vi "voltech4_test.vi"() -> ()   [LabVIEW 2015]
uses:
  <instrlib>/Voltech PM1000+/Voltech PM1000+.lvlib
  <vilib>/Utility/file.llb/Write To Spreadsheet File (string).vi
  <instrlib>/Voltech PM1000+/Public/Configure/Configure Measurements (Normal).vi
panel:
  out "error3":string
  out "output 3":string
  out "String 3":string
  out "output before loop":string
  out "error before":string
  in  "Minutes per test":dbl
  in  "FOLDER NAME":string
  in  "HOW MANY TEST":i32
  in  "Name of File":string
  in  "VISA resource name 2":refnum<visa-resource-name>
  out "Current Data Point":i32
  in  "stop":bool
  out "VRMS":dbl[](graph)
  in  "Normal Measurements":i32[](listbox)=[0, 1, 2, 3, 4, 5, 6]
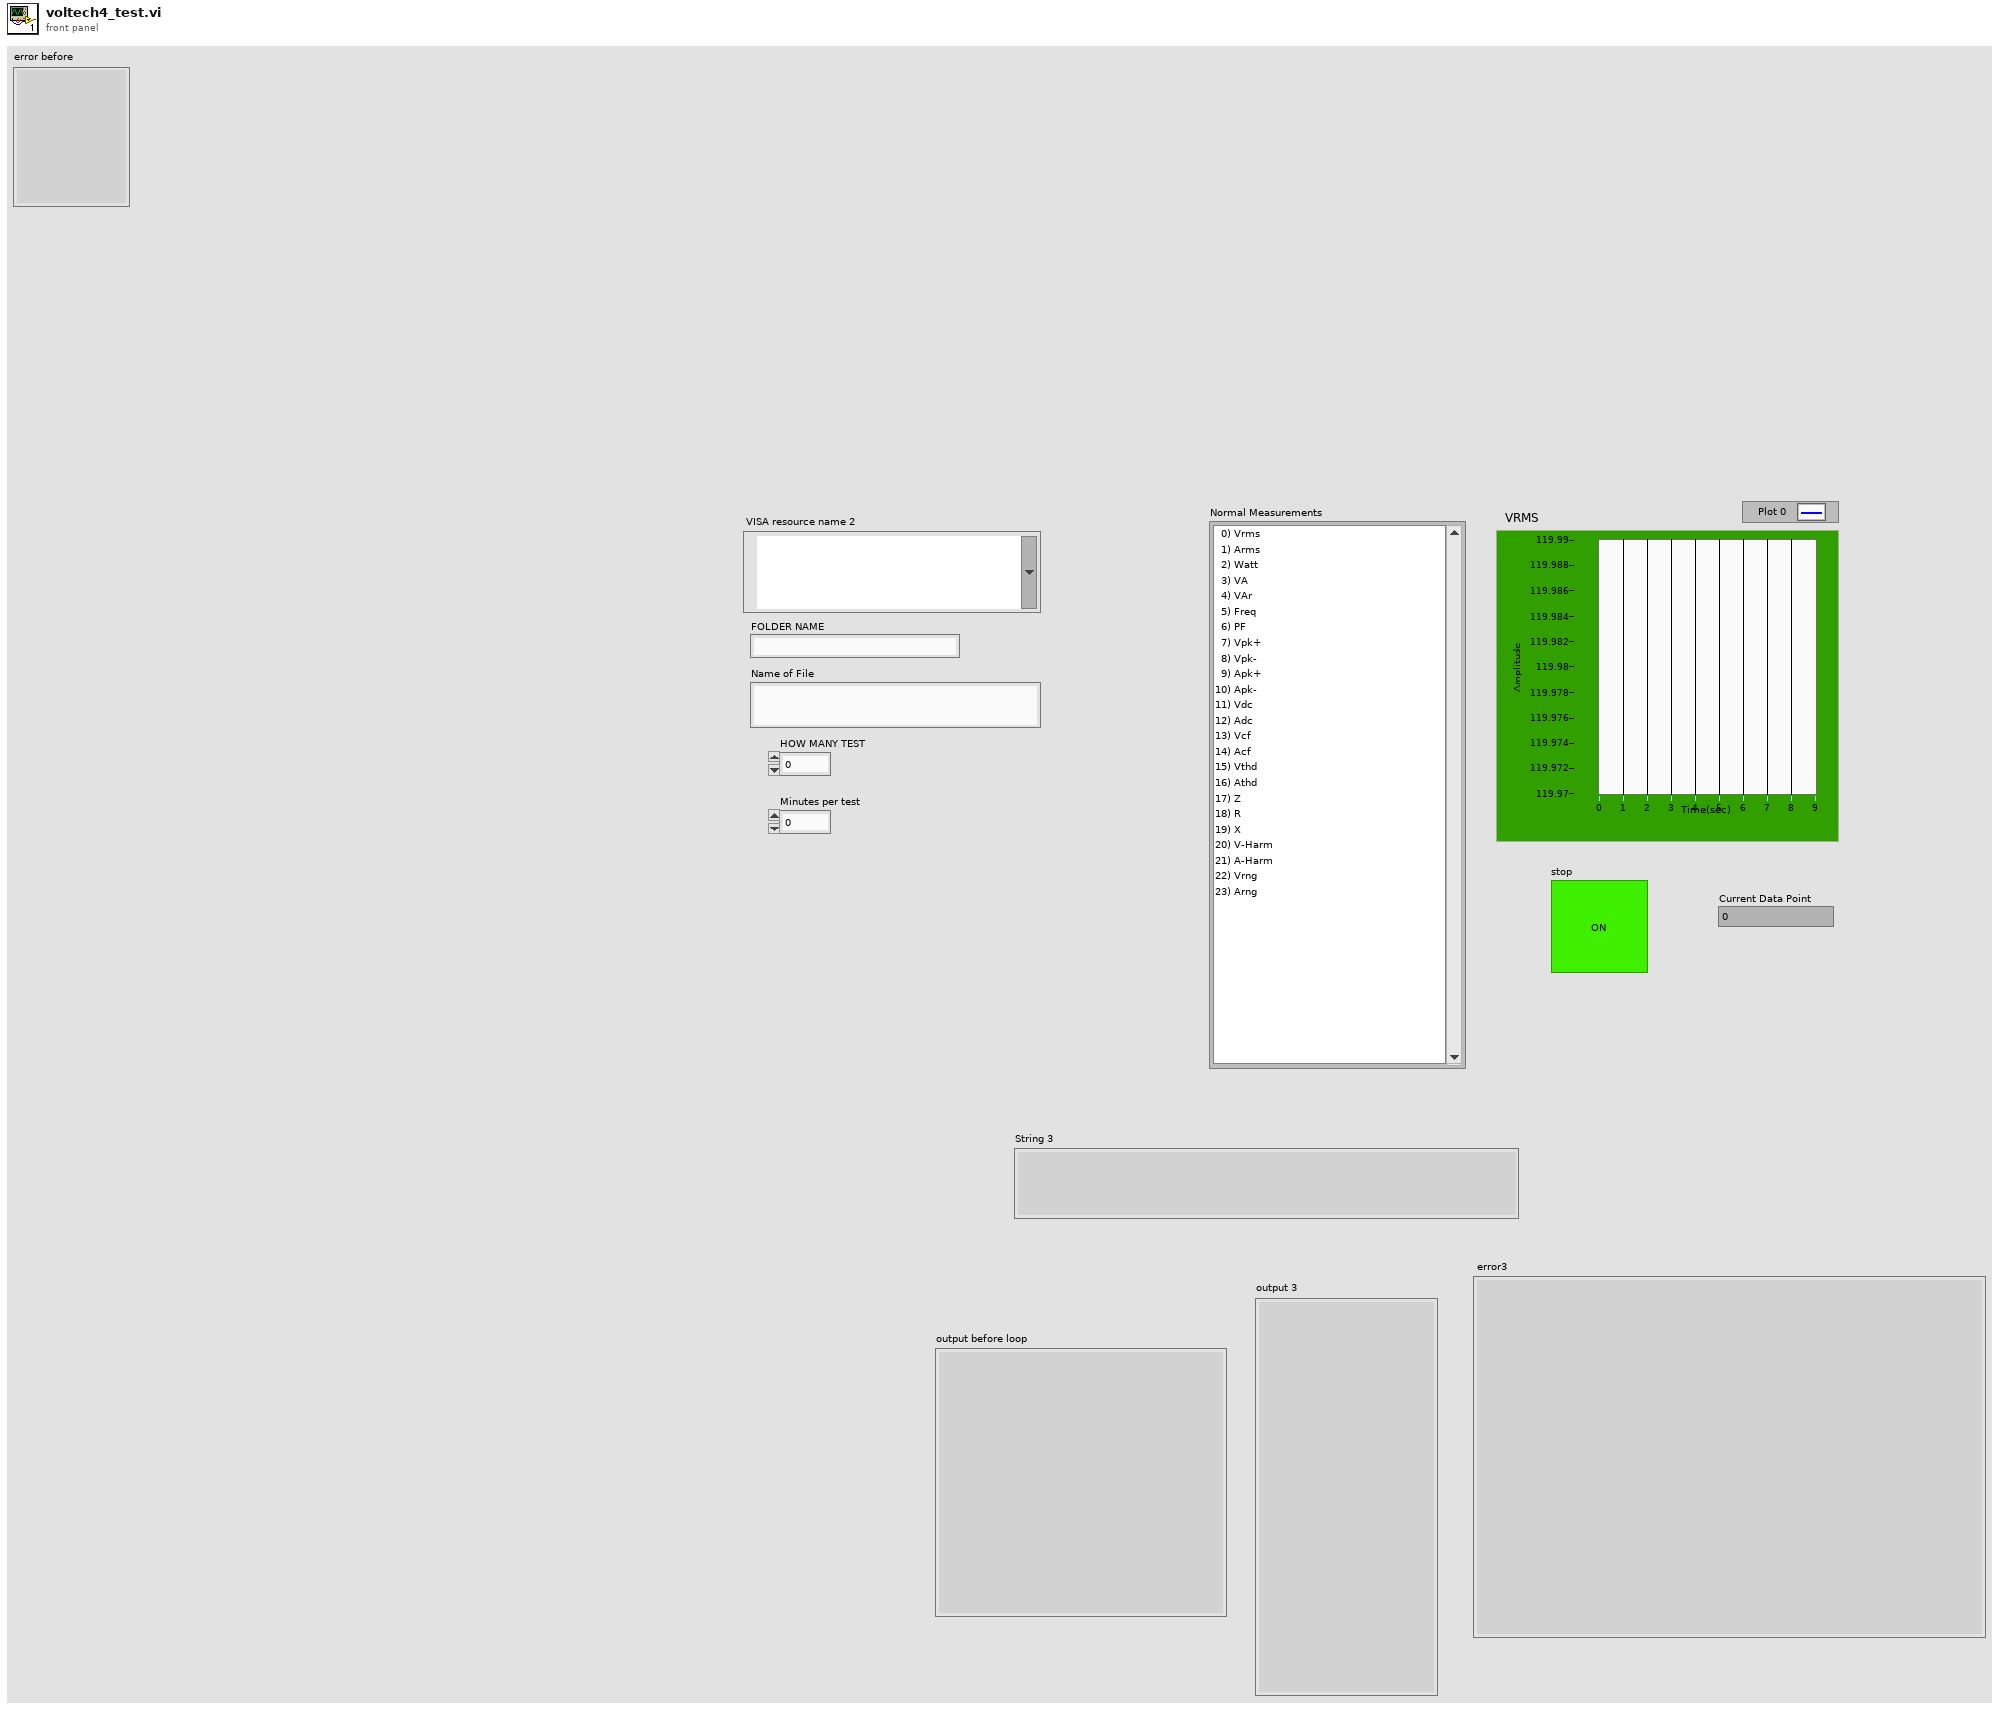
[diagram p1: front panel]
types:
  T1 = enum16{"open", "replace", "create", "open or create", "replace or create", "replace or create with confirmation"}
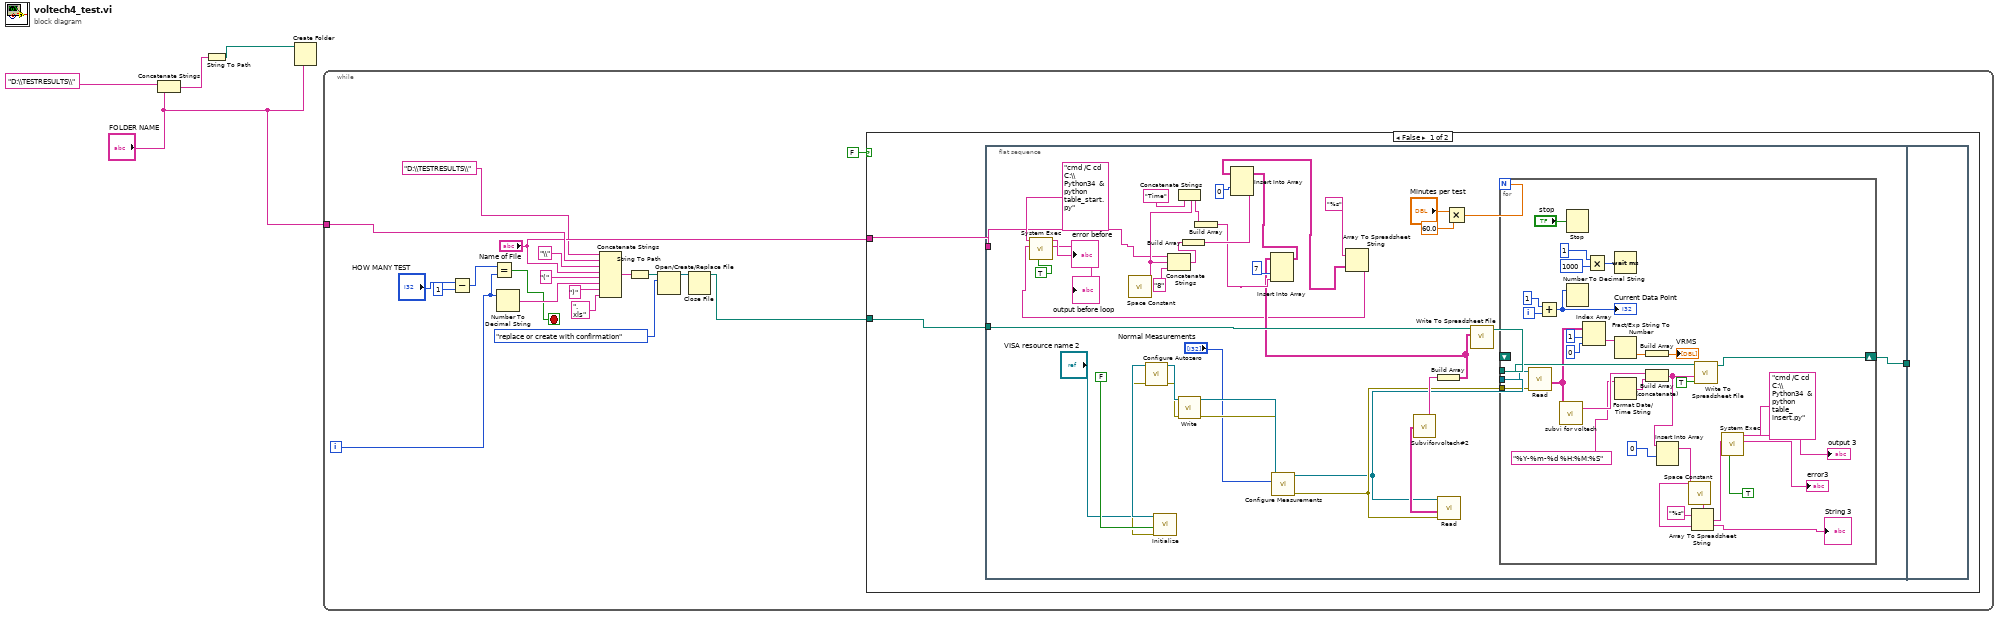
[diagram p0: block diagram]
diagram:
  n1 = Concatenate Strings("D:\\TESTRESULTS\\" ("string"), "FOLDER NAME") -> (w2:string)
  n2 = String To Path(string=w2) -> (path=w1:path)
  n3 = Create Folder(prompt (Create Folder)="FOLDER NAME", path (use dialog)=w1) -> ()  [unwired: 1 in, 3 out]
  n4 = while {
    tunnel: "FOLDER NAME" -> [w10]
    i -> [w11]
    stop <- w12 stop-if-true
    n5 = Subtract(x="HOW MANY TEST", y=1) -> (x-y=w7:i32)
    n6 = Equal?(x=w7, y=w11) -> (x = y?=w12:bool)
    n7 = Number To Decimal String(number=w11) -> (decimal integer string=w16:string)  [unwired: 1 in]
    n8 = Concatenate Strings("D:\\TESTRESULTS\\" ("string"), w10, "\\" ("string"), "Name of File", "(" ("string"), w16, ")" ("string"), ".xls" ("string")) -> (w20:string)
    n9 = String To Path(string=w20) -> (path=w21:path)
    n10 = Open/Create/Replace File(file path (use dialog)=w21, operation (0:open)=T1."replace or create with confirmation") -> (refnum out=w19:refnum<file>)  [unwired: 4 in, 2 out]
    n11 = Close File(refnum=w19) -> (path=w13:path)  [unwired: 1 in, 1 out]
    n12 = case shown="False" FALSE {
      tunnel: w13 -> [w26 _]
      tunnel: "Name of File" -> [w24 _]
      frame False {
        n13 = flat-sequence {
          tunnel: w26 -> [w54]
          tunnel: [w60] -> w25
          tunnel: w24 -> [w30]
          tunnel: w25 -> [_]
          frame #0 {
            n14 = call <vilib>:"Space Constant.vi"() -> ("String"=w35:string)
            n15 = call <instrlib>:"Initialize.vi"("Reset (True)"=FALSE, "VISA resource name"="VISA resource name 2") -> ("error out"=w62:errorcluster, "VISA resource name out"=w63:refnum<visa-resource-name>)  [unwired: 8 in]
            n16 = call <instrlib>:"Configure Autozero.vi"("error in (no error)"=w62, "VISA resource name"=w63) -> ("error out"=w58:errorcluster, "VISA resource name out"=w59:refnum<visa-resource-name>)  [unwired: 8 in]
            n17 = Concatenate Strings(w30, w35, "8") -> (w37:string)
            n18 = Concatenate Strings("Time", w35) -> (w32:string)
            n19 = call <instrlib>:"Write.vi"("error in (no error)"=w58, "VISA resource name"=w59) -> ("error out"=w56:errorcluster, "VISA resource name out"=w57:refnum<visa-resource-name>)  [unwired: 8 in]
            n20 = Build Array(w37) -> (w38:string[])
            n21 = Build Array(w32) -> (w33:string[])
            n22 = call-poly <instrlib>:"Configure Measurements.vi"("error in (no error)"=w56, "Normal Measurements"="Normal Measurements", "VISA resource name"=w57) -> ("error out"=w50:errorcluster, "VISA resource name out"=w49:refnum<visa-resource-name>)  [unwired: 7 in]
            n23 = call <instrlib>:"Read.vi"("error in (no error)"=w50, "VISA resource name"=w49) -> ("Measurement Results"=w51:string[][])  [unwired: 7 in, 2 out]
            n24 = call "Subviforvoltech#2.vi"("Measurement Results 2"=w51) -> ("Array"=w55:string[])
            n25 = Build Array(w55) -> (w29:string[][])
            n26 = Insert Into Array(array=w29, index (col)=7, new element=w33) -> (w40:string[][])  [unwired: 1 in]
            n27 = Insert Into Array(array=w40, index (col)=0, new element=w38) -> (w27:string[][])  [unwired: 1 in]
            n28 = Array To Spreadsheet String(array=w27, 3:"%s") -> (spreadsheet string=w28:string)  [unwired: 1 in]
            n29 = call <vilib>:"System Exec.vi"("run minimized? (F)"=TRUE, "standard input"=w28, "command line"="cmd /C cd C:\\Python34  & python table_start.py") -> ("standard error"=→"output before loop":string, "standard output"=→"error before":string)  [unwired: 5 in, 2 out]
            n30 = Multiply(x="Minutes per test", y=60.0) -> (x*y=w48:dbl)
            n31 = call-poly <vilib>:"Write To Spreadsheet File.vi"("2D data"=w29, "file path (dialog if empty)"=w54) -> ("new file path (Not A Path if cancelled)"=w53:path)  [unwired: 6 in]
            n32 = for {
              N: w48 -> [_]
              tunnel: w53 -> [w90]
              shift-right: [w88] -> w60
              shift-left: _ -> [_]
              tunnel: w49 -> [w86]
              tunnel: w50 -> [w85]
              i -> [w92]
              n33 = call <instrlib>:"Read.vi"("error in (no error)"=w85, "VISA resource name"=w86) -> ("Measurement Results"=w77:string[][])  [unwired: 7 in, 2 out]
              n34 = Add(x=1, y=w92) -> (x+y=w93:i32)
              "Current Data Point" <- w93
              n35 = call "subvi for voltech.vi"("Measurement Results 2"=w77) -> ("Array"=w87:string[])  [unwired: 6 in]
              n36 = Stop(stop? (T)="stop") -> ()
              n37 = Number To Decimal String(number=w93) -> ()  [unwired: 1 in, 1 out]
              n38 = Index Array(array=w77, index (row)=1, index (col)=0 ("disabled index (col)")) -> (element=w80:string)
              n39 = Multiply(x=u32 1 ("Interval of Data Collection (sec)"), y=u32 1000) -> (x*y=w94:u32)
              n40 = Wait (ms)(milliseconds to wait=w94) -> ()  [unwired: 1 out]
              n41 = Fract/Exp String To Number(string=w80) -> (number=w76:dbl)  [unwired: 3 in, 1 out]
              n42 = Format Date/Time String(time format string (%c)="%Y-%m-%d %H:%M:%S") -> (date/time string=w83:string)  [unwired: 2 in]
              n43 = Build Array(w76) -> (→"VRMS":dbl[])
              n44 = Build Array (concatenate)(w87, w83) -> (w68:string[])
              n45 = Insert Into Array(array=w68, index=0) -> (w73:string[])  [unwired: 1 in]
              n46 = call <vilib>:"Space Constant.vi"() -> ("String"=w75:string)
              n47 = Array To Spreadsheet String(delimiter (Tab)=w75, array=w73, 3:"%s") -> (spreadsheet string=w66:string)
              "String 3" <- w66
              n48 = call-poly <vilib>:"Write To Spreadsheet File.vi"("append to file? (new file:F)"=TRUE, "1D data"=w68, "file path (dialog if empty)"=w90) -> ("new file path (Not A Path if cancelled)"=w88:path)  [unwired: 5 in]
              n49 = call <vilib>:"System Exec.vi"("run minimized? (F)"=TRUE, "standard input"=w66, "command line"="cmd /C cd C:\\Python34  & python table_insert.py") -> ("standard error"=→"error3":string, "standard output"=→"output 3":string)  [unwired: 5 in, 2 out]
            }
          }
          frame #1 {
          }
        }
      }
      frame True {
      }
    }
  }
